vi "scanXY.vi"(5 "Activar movimiento en Z":bool, 6 "Error In":errorcluster, 7 "Micras en Z":dbl, 8 "Activar movimiento en Y":bool, 9 "Activar movimiento en X":bool, 10 "Micras en Y":dbl, 11 "Micras en X":dbl) -> (4 "Error Out":errorcluster)   [LabVIEW 2018]
uses:
  <vilib>/Instr/_visa.llb/VISA Configure Serial Port (Instr).vi
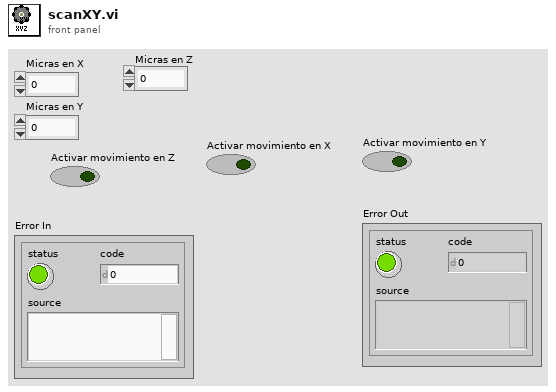
[diagram p1: front panel]
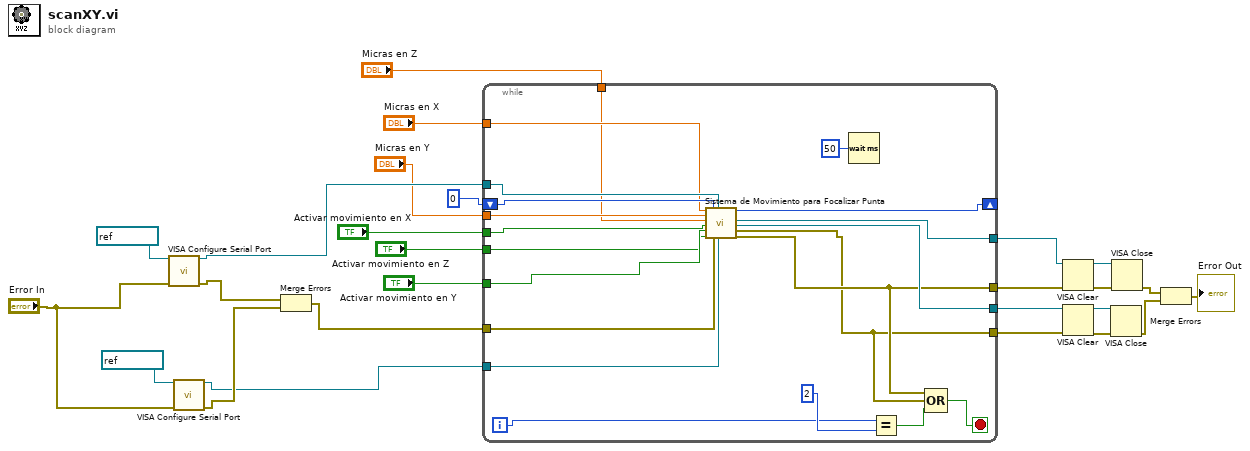
[diagram p0: block diagram]
diagram:
  n1 = call-poly "VISA Configure Serial Port"("VISA resource name"=refnum<visa-resource-name> "COM7", "error in (no error)"="Error In") -> ("VISA resource name out"=w19:refnum<visa-resource-name>, "error out"=w22:errorcluster)  [unwired: 12 in]
  n2 = call-poly "VISA Configure Serial Port"("VISA resource name"=refnum<visa-resource-name> "COM6", "error in (no error)"="Error In") -> ("VISA resource name out"=w20:refnum<visa-resource-name>, "error out"=w21:errorcluster)  [unwired: 12 in]
  n3 = Merge Errors(w22, w21) -> (w18:errorcluster)
  n4 = while {
    shift-right: [w33] -> _
    shift-left: 0 -> [w46]
    tunnel: w20 -> [w45]
    tunnel: w19 -> [w44]
    tunnel: w18 -> [w43]
    tunnel: [w42] -> w10
    tunnel: [w41] -> w9
    tunnel: [w38] -> w8
    tunnel: [w37] -> w7
    tunnel: "Micras en X" -> [w35]
    tunnel: "Micras en Y" -> [w34]
    tunnel: "Micras en Z" -> [w31]
    tunnel: "Activar movimiento en X" -> [w30]
    tunnel: "Activar movimiento en Y" -> [w29]
    tunnel: "Activar movimiento en Z" -> [w28]
    i -> [w32]
    stop <- w39 stop-if-true
    n5 = call "Sistema de Movimiento para Focalizar Punta.vi"("Micras en X"=w35, "Micras en Y"=w34, "Micras en Z"=w31, "Activar movimiento en X"=w30, "Activar movimiento en Y"=w29, "Activar movimiento en Z"=w28, "Caso de Entrada"=w46, "error in"=w43, "VISA Micro XY"=w44, "VISA Micro Z"=w45) -> ("Caso de salida"=w33:i32, "VISA resource name out"=w42:refnum<visa-resource-name>, "VISA resource name out 2"=w41:refnum<visa-resource-name>, "error out Z"=w37:errorcluster, "error out XY"=w38:errorcluster)  [unwired: 5 in]
    n6 = Wait (ms)(milliseconds to wait=u32 50) -> ()  [unwired: 1 out]
    n7 = Equal?(x=w32, y=2 ("x")) -> (x = y?=w40:bool)
    n8 = Compound Arithmetic op=OR(w38, w37, w40) -> (w39:bool)
  }
  n9 = VISA Clear(VISA resource name=w10, error in (no error)=w8) -> (VISA resource name out=w16:refnum<visa-resource-name>, error out=w17:errorcluster)
  n10 = VISA Clear(VISA resource name=w9, error in (no error)=w7) -> (VISA resource name out=w15:refnum<visa-resource-name>, error out=w14:errorcluster)
  n11 = VISA Close(VISA resource name=w15, error in (no error)=w14) -> (error out=w12:errorcluster)
  n12 = VISA Close(VISA resource name=w16, error in (no error)=w17) -> (error out=w13:errorcluster)
  n13 = Merge Errors(w13, w12) -> (→"Error Out":errorcluster)
